vi "OtherNumerics.vi"() -> ()   [LabVIEW 2020]
panel:
  out "x-y*floor(x/y)":dbl
  out "number (0 to 1)":dbl
  out "Numeric":dbl=2.220446049250313e-16
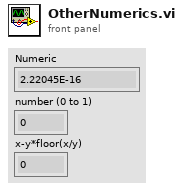
[diagram p1: front panel]
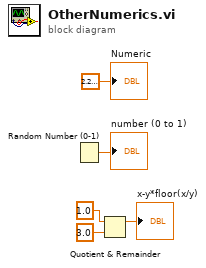
[diagram p0: block diagram]
diagram:
  n1 = Random Number (0-1)() -> (number: 0 to 1=→"number (0 to 1)":dbl)
  n2 = Quotient & Remainder(x=1.0, y=3.0) -> (x-y*floor(x/y)=→"x-y*floor(x/y)":dbl)  [unwired: 1 out]
  "Numeric" <- 2.220446049250313e-16
